vi "S7_Read_Write_Data_TCP.vi"(0 "TCP Connection Ref":refnum<k5>, 1 "Read / Write":u8(ring)=4 items=["Read"=4, "Write"=5], 5 "Address Areas":u8(ring)=128 format="%02x" items=["I/O (P)"=128, "Input (I)"=129, "Output (Q)"=130, "Bit Memory (M)"=131, "Data (DB)"=132, "Instance Data (DI)"=133, "Local Data (L)"=134, "Predecessor Local Data (VL)"=135], 7 "Start Address (bytes)":u32=131, 9 "Data Block #":u16=1, 11 "error in":errorcluster, 12 "Write Data":u8 format="%02x", 13 "Length (bytes)":u16=1, 14 "Timeout":u32=1000) -> (4 "TCP Connection Ref Out":refnum<k5>, 6 "Data Valid":bool, 8 "Comm Error":u16, 10 "Data Read":u8[](array[numeric]), 15 "error out":errorcluster)   [LabVIEW 2018, in "S7 TCP.lvlib"]
uses:
  S7 TCP.lvlib
panel:
  # "Max Length = 222\n(corresponds to total\nPDU length of 240; 18\nvalues in PDU & data\nheader)"
  # "Data Block only valid\nwhen reading / writing \n\"Data (DB)\" Address Area"
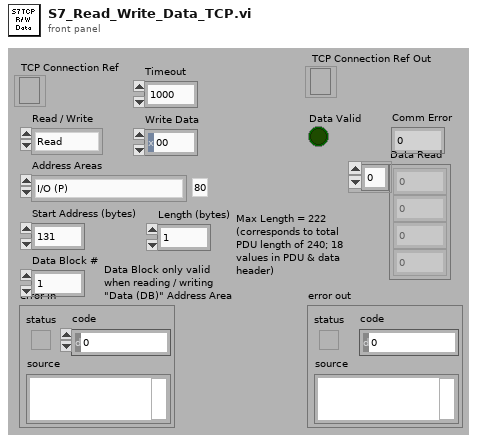
[diagram p1: front panel]
types:
  T1 = enum16{"Standard", "Buffered", "CRLF", "Immediate"}
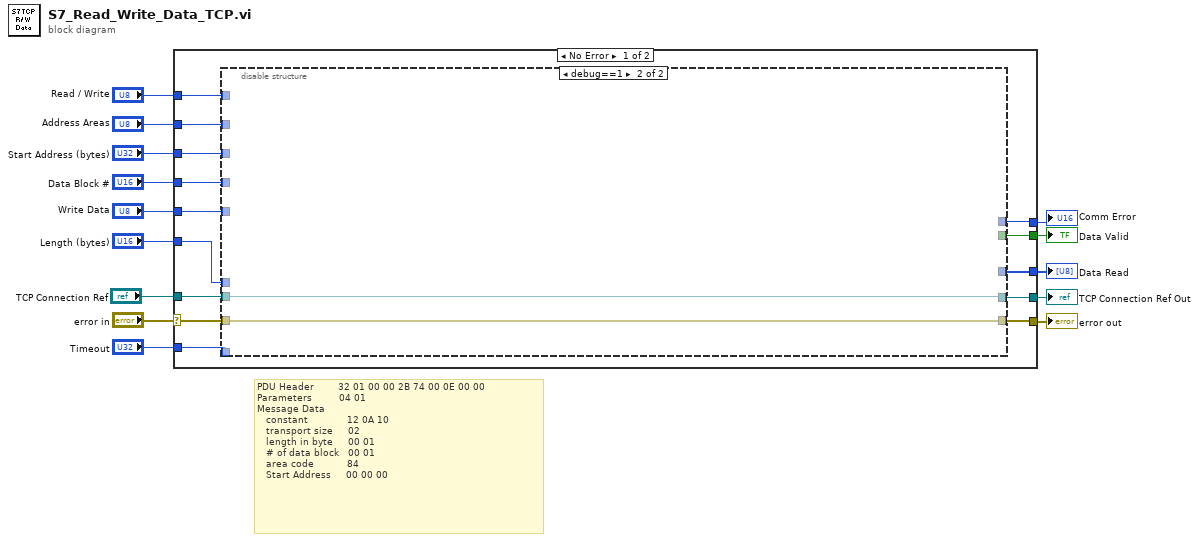
[diagram p0: block diagram]
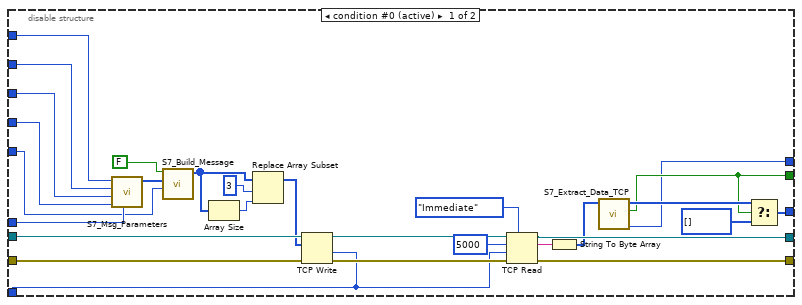
[diagram p2: hidden frame]
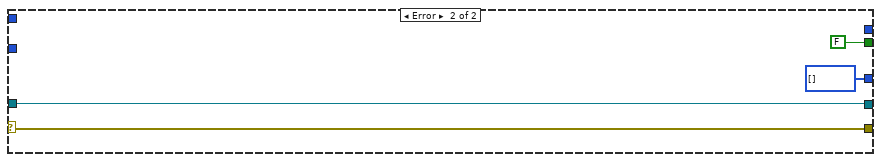
[diagram p3: hidden frame]
diagram:
  # "PDU Header        32 01 00 00 2B 74 00 0E 00 00 \nParameters         04 01 \nMessage Data       \n   constant             12 0A 10\n   transport size     02\n   length in byte     00 01\n   # of data block   00 01\n   area code           84\n   Start Address     00 00 00"
  n1 = case shown="No Error" "error in" {
    selector: "error in" -> [w21 w61]
    tunnel: "TCP Connection Ref" -> [w22 w62]
    tunnel: "Timeout" -> [w18 _]
    tunnel: "Length (bytes)" -> [w28 _]
    tunnel: "Write Data" -> [w27 _]
    tunnel: "Data Block #" -> [w26 _]
    tunnel: "Start Address (bytes)" -> [w25 _]
    tunnel: "Address Areas" -> [w24 _]
    tunnel: "Read / Write" -> [w16 _]
    tunnel: [w20 w62] -> w2
    tunnel: [w19 w61] -> w7
    tunnel: [w17 u8[] [] ("f")] -> w6
    tunnel: [w23 FALSE ("Data Valid")] -> w5
    tunnel: [w15 _] -> w1
    frame No Error {
      n2 = disable-structure shown="debug==1" {
        disable-tunnel: w28 -> [w55 _]
        disable-tunnel: w27 -> [w54 _]
        disable-tunnel: w26 -> [w53 _]
        disable-tunnel: w25 -> [w52 _]
        disable-tunnel: w24 -> [w51 _]
        disable-tunnel: [w47 _] -> w23
        disable-tunnel: w22 -> [w46 w57]
        disable-tunnel: w21 -> [w45 w58]
        disable-tunnel: [w42 w57] -> w20
        disable-tunnel: [w41 w58] -> w19
        disable-tunnel: w18 -> [w39 _]
        disable-tunnel: [w35 _] -> w17
        disable-tunnel: w16 -> [w34 _]
        disable-tunnel: [w29 _] -> w15
        frame condition #0 (active) {
          n3 = call "S7_Msg_Parameters.vi"("Length (bytes)"=w55, "Data Block #"=w53, "Start Address (bytes)"=w52, "Address Areas"=w51, "Read / Write"=w34) -> ("Message Parameters"=w56:u8[])  [unwired: 6 out]
          n4 = call "S7_Build_Message.vi"("Write Data"=w54, "Parameters"=w56, "Exchange PDU"=FALSE) -> ("S7 Ethernet Data"=w30:u8[])  [unwired: 8 out]
          n5 = Array Size(array=w30) -> (size(s)=w31:i32)
          n6 = Replace Array Subset(array=w30, new element=w31, index=3) -> (w33:u8[])
          n7 = TCP Write(connection ID=w46, data in=w33, error in (no error)=w45, 9:w39) -> (connection ID out=w44:refnum<k5>, error out=w43:errorcluster)  [unwired: 1 out]
          n8 = TCP Read(connection ID=w44, bytes to read=5000, error in (no error)=w43, 7:T1."Immediate" ("mode (standard)"), 9:w39) -> (connection ID out=w42:refnum<k5>, data out=w40:string, error out=w41:errorcluster)
          n9 = String To Byte Array(string=w40) -> (unsigned byte array=w36:u8[])
          n10 = call "S7_Extract_Data_TCP.vi"("Data Recieved"=w36) -> ("Error"=w29:u16, "Data Valid"=w47:bool, "Data"=w49:u8[])  [unwired: 8 out]
          n11 = Select(t=w49, s=w47, f=u8[] []) -> (s? t:f=w35:u8[])
        }
        frame condition #1 {
        }
      }
    }
    frame Error {
    }
  }
  "error out" <- w7
  "Data Read" <- w6
  "Data Valid" <- w5
  "TCP Connection Ref Out" <- w2
  "Comm Error" <- w1
